vi "filter_frequency_strain_9215_v2.vi"() -> ()   [LabVIEW 2014]
uses:
  <vilib>/rvi/Analysis/host/Butterworth/config/Butterworth Filter Order.ctl
  <vilib>/rvi/Analysis/host/Butterworth/config/Butterworth Filter Type.ctl
  <vilib>/FPGAPlugInAG/cRIO-9039/niLvFpga_Open_cRIO-9039.vi
  <vilib>/rvi/interface/common/dynamic/niFpgaDynamicAddResources.vi
  <vilib>/rvi/Analysis/host/Butterworth/config/BwScaledCoefficients.vi
  <vilib>/Utility/error.llb/Error Cluster From Error Code.vi
  <vilib>/rvi/errors/niLvFpgaAdjustHostInterfaceError.vi
  <vilib>/FPGAPlugInAG/Dynamic/niLvFpga_Close_Dynamic.vi
  <vilib>/rvi/interface/nirviOpenFPGA/nirviOpenFPGA.xnode
  FPGA Bitfiles/test0304_FPGATarget_strain9215v2_tBjd64kN5cY.lvbitx
  strain_9215_v2.vi
  <vilib>/rvi/Analysis/host/Butterworth/XNode/ButterworthCoefficients.xnode
  <vilib>/rvi/interface/nirviReadWriteControl/nirviReadWriteControl.xnode
  <vilib>/rvi/interface/nirviCloseFPGA/nirviCloseFPGA.xnode
  NiFpgaLv.dll
  <vilib>/rvi/interface/Simulation/niFpgaSimulationCallBeginRW.vi
  <vilib>/rvi/Analysis/host/Public/NI_FpgaMspHost.lvlib
panel:
  in  "stop":bool
  in  "sample rate (S/s)":dbl=50000.0
  in  "fcu_p_Avg2 (Hz)":dbl=1000.0
  in  "fcu_p_Avg4 (Hz)":dbl=1000.0
  in  "fcu_p_Avg8 (Hz)":dbl=1000.0
  in  "fcu_y_Avg2 (Hz)":dbl=1000.0
  in  "fcu_y_Avg4 (Hz)":dbl=1000.0
  in  "fcu_y_Avg8 (Hz)":dbl=1000.0
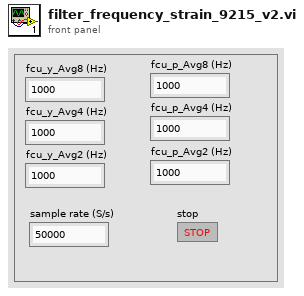
[diagram p1: front panel]
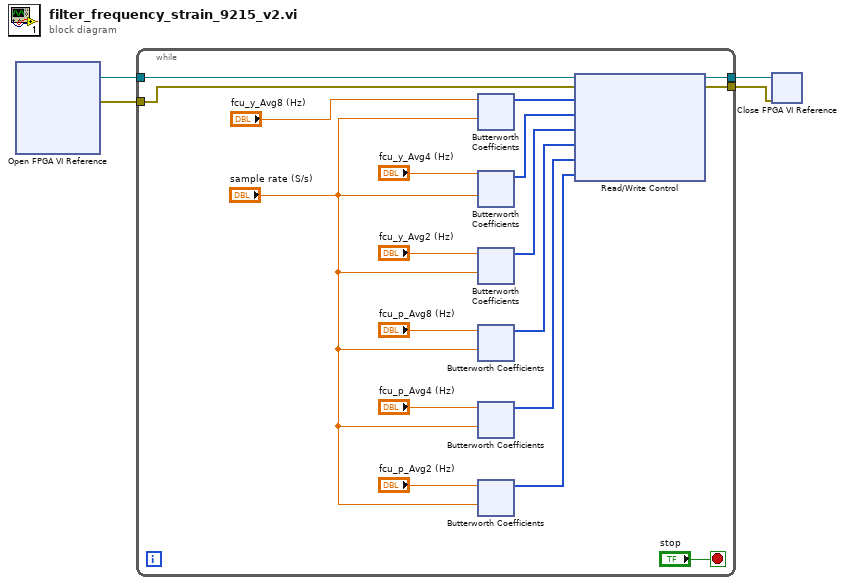
[diagram p0: block diagram]
diagram:
  n1 = xnode "Open FPGA VI Reference"() -> ("FPGA VI Reference Out"=w4:refnum<k20>, "error out"=w3:errorcluster)  [unwired: 2 in]
  n2 = while {
    tunnel: w4 -> [w22]
    tunnel: w3 -> [w19]
    tunnel: [w21] -> w2
    tunnel: [w20] -> w1
    stop <- "stop" stop-if-true
    n3 = xnode "Butterworth Coefficients"("cutoff frequency (Hz)"="fcu_y_Avg8 (Hz)", "sample rate (S/s)"="sample rate (S/s)") -> ("scaled coefficients"=w18:i32[])  [unwired: 1 in, 1 out]
    n4 = xnode "Butterworth Coefficients"("cutoff frequency (Hz)"="fcu_y_Avg4 (Hz)", "sample rate (S/s)"="sample rate (S/s)") -> ("scaled coefficients"=w17:i32[])  [unwired: 1 in, 1 out]
    n5 = xnode "Butterworth Coefficients"("cutoff frequency (Hz)"="fcu_y_Avg2 (Hz)", "sample rate (S/s)"="sample rate (S/s)") -> ("scaled coefficients"=w16:i32[])  [unwired: 1 in, 1 out]
    n6 = xnode "Butterworth Coefficients"("cutoff frequency (Hz)"="fcu_p_Avg8 (Hz)", "sample rate (S/s)"="sample rate (S/s)") -> ("scaled coefficients"=w15:i32[])  [unwired: 1 in, 1 out]
    n7 = xnode "Butterworth Coefficients"("cutoff frequency (Hz)"="fcu_p_Avg4 (Hz)", "sample rate (S/s)"="sample rate (S/s)") -> ("scaled coefficients"=w14:i32[])  [unwired: 1 in, 1 out]
    n8 = xnode "Butterworth Coefficients"("cutoff frequency (Hz)"="fcu_p_Avg2 (Hz)", "sample rate (S/s)"="sample rate (S/s)") -> ("scaled coefficients"=w13:i32[])  [unwired: 1 in, 1 out]
    n9 = xnode "Read/Write Control"("FPGA VI Reference In"=w22, "error in"=w19, "Strain_y Avg8 coeff."=w18, "Strain_y Avg4 coeff."=w17, "Strain_y Avg2 coeff."=w16, "Strain_p Avg8 coeff."=w15, "Strain_p Avg4 coeff."=w14, "Strain_p Avg2 coeff."=w13) -> ("FPGA VI Reference Out"=w21:refnum<k20>, "error out"=w20:errorcluster)
  }
  n10 = xnode "Close FPGA VI Reference"("FPGA VI Reference In"=w2, "error in"=w1) -> ()  [unwired: 1 out]
